vi "Modify JSON Text.vi"(10 "Parameter and Value":string, 11 "JSONtextin":string) -> (3 "JSONtextout":string="{\n    \"SMUResourceName\": \"SMU\",\n    \"SMUChannels\": \"0\",\n\t\"SMUSourceMode_Sequence\": 1021,\n\t\"SMUOutputFunction_DCCurrent\": 1007,\n    \"SMUSourceTransientResponse_Fast\": 1039,\n    \"SMUCurrent\": 1.0,\n    \"SMUCurrentLevelRange\": 1.0,\n    \"SMUMeasurementSense_Local\": 1008,\n    \"SMUMeasurementApertureTime\": 0.010,\n    \"SMUSourceAdvancedSourceDelay\": 0.000100,\n    \"SMUVoltage\": 6,\n    \"SMUSourceAdvancedSequenceLoopCount\": 571,\n    \"SMUMeasurementAdvancedDCNoiseRejection_Normal\": 1044,\n\t\"SMUSequenceName\": \"MySequence\",\n\t\"SMUStep1_Source_DCCurrent_CurrentLevel\": 1150009,\n\t\"SMUStep2_Measurement_ApertureTime\": 1150058,\n\t\"SMUStep3_Source_Advanced_SourceDelay\": 1150051,\n\t\"SMUSequenceNumberOfSteps\": 3,\n\t\"SMUTriggerFromSwitch_StartDigitalEdge\": \"/SMU/PXI_Trig1\",\n\t\"SMUTriggerFromSwitch_SequenceAdvanceDigitalEdge\": \"/SMU/PXI_Trig1\",\n\t\"SMUTriggerToDMM_SourceCompleteEvent\": 1030,\n\t\"SMUTriggerToDMM_SourceCompleteEvent_Value\": \"/SMU/PXI_Trig2\",\n\t\"SMUTriggerToSwitch_SequenceIterationCompleteEvent\": 1032,\n\t\"SMUTriggerToDMM_SequenceIterationCompleteEvent_Value\": \"/SMU/PXI_Trig0\",\n\t\n\t\"Switch1ResourceName\": \"2526_1\",\n\t\"Switch1Topology\": \"2526/2-Wire 79x1 Mux\",\n\t\"Switch1ScanList\": \"ch70:75->com\",\n\t\n\t\"Switch2ResourceName\": \"SwitchBlock1Dev1\",\n\t\"Switch2Topology\": \"Configured Topology\",\n\t\"Switch2ScanList\": \"[c2->card1r2->c26], [c3->card1r3->c27]; [c6->card1r2->c26], [c7->card1r3->c27]; [c10->card1r2->c26], [c11->card1r3->c27]; [c14->card1r2->c26], [c15->card1r3->c27]; [c18->card1r2->c26], [c19->card1r3->c27]; [c22->card1r2->c26], [c23->card1r3->c27];\"\n}")   [LabVIEW 2019]
panel:
  in  "Parameter and Value (for unit testing)":string[](array[string])=["SETCONF=SMUResourceName[[CONFPARAM]]=SMU", "SETCONF=SMUChannels[[CONFPARAM]]=0", "SETCONF=SMUSourceMode_Sequence[[CONFPARAM]]=1021", "SETCONF=SMUOutputFunction_DCCurrent[[CONFPARAM]]=1007", "SETCONF=SMUSourceTransientResponse_Fast[[CONFPARAM]]=1039", "SETCONF=SMUCurrent[[CONFPARAM]]=1.0", "SETCONF=SMUCurrentLevelRange[[CONFPARAM]]=1.0", "SETCONF=SMUMeasurementSense_Local[[CONFPARAM]]=1008", "SETCONF=SMUMeasurementApertureTime[[CONFPARAM]]=0.010", "SETCONF=SMUSourceAdvancedSourceDelay[[CONFPARAM]]=0.000100", "SETCONF=SMUVoltage[[CONFPARAM]]=6", "SETCONF=SMUSourceAdvancedSequenceLoopCount[[CONFPARAM]]=571", "SETCONF=SMUMeasurementAdvancedDCNoiseRejection_Normal[[CONFPARAM]]=1044", "SETCONF=SMUSequenceName[[CONFPARAM]]=MySequence", "SETCONF=SMUStep1_Source_DCCurrent_CurrentLevel[[CONFPARAM]]=1150009", "SETCONF=SMUStep2_Measurement_ApertureTime[[CONFPARAM]]=1150058", "SETCONF=SMUStep3_Source_Advanced_SourceDelay[[CONFPARAM]]=1150051", "SETCONF=SMUSequenceNumberOfSteps[[CONFPARAM]]=3", "SETCONF=SMUTriggerFromSwitch_StartDigitalEdge[[CONFPARAM]]=/SMU/PXI_Trig1", "SETCONF=SMUTriggerFromSwitch_SequenceAdvanceDigitalEdge[[CONFPARAM]]=/SMU/PXI_Trig1", "SETCONF=SMUTriggerToDMM_SourceCompleteEvent[[CONFPARAM]]=1030", "SETCONF=SMUTriggerToDMM_SourceCompleteEvent_Value[[CONFPARAM]]=/SMU/PXI_Trig2", "SETCONF=SMUTriggerToSwitch_SequenceIterationCompleteEvent[[CONFPARAM]]=1032", "SETCONF=SMUTriggerToDMM_SequenceIterationCompleteEvent_Value[[CONFPARAM]]=/SMU/PXI_Trig0", "SETCONF=Switch1ResourceName[[CONFPARAM]]=2526_1", "SETCONF=Switch1Topology[[CONFPARAM]]=2526/2-Wire 79x1 Mux", "SETCONF=Switch1ScanList[[CONFPARAM]]=ch70:75->com", "SETCONF=Switch2ResourceName[[CONFPARAM]]=SwitchBlock1Dev1", "SETCONF=Switch2Topology[[CONFPARAM]]=Configured Topology", "SETCONF=Switch2ScanList[[CONFPARAM]]=[c2->card1r2->c26], [c3->card1r3->c27]; [c6->card1r2->c26], [c7->card1r3->c27]; [c10->card1r2->c26], [c11->card1r3->c27]; [c14->card1r2->c26], [c15->card1r3->c27]; [c18->card1r2->c26], [c19->card1r3->c27]; [c22->card1r2->c26], [c23->card1r3->c27];", "SETCONF=DMMResourceName[[CONFPARAM]]=DMM", "SETCONF=DMMFunction_DCVolts[[CONFPARAM]]=0", "SETCONF=DMMResolution[[CONFPARAM]]=0.1", "SETCONF=DMMRange[[CONFPARAM]]=0.1", "SETCONF=DMMTriggerSource_TTL2[[CONFPARAM]]=4", "SETCONF=DMMTriggerSlope_RisingEdge[[CONFPARAM]]=0", "SETCONF=DMMSampleTrigger_TTL2[[CONFPARAM]]=4", "SETCONF=DMMSampleCount[[CONFPARAM]]=0", "SETCONF=DMMSampleTriggerSlope_RisingEdge[[CONFPARAM]]=0", "SETCONF=DMMApertureTimeUnits_Seconds[[CONFPARAM]]=0", "SETCONF=DMMApertureTime[[CONFPARAM]]=0.010", "SETCONF=DMMNumberOfAverages[[CONFPARAM]]=1", "SETCONF=DMMAutoZero_Off[[CONFPARAM]]=0", "SETCONF=DMMADCCalibration_Off[[CONFPARAM]]=0", "SETCONF=DMMSettleTime[[CONFPARAM]]=0.0001", "SETCONF=DMMControlAction_Commit[[CONFPARAM]]=0", "SETCONF=ApplicationNumberOfWeldChannels[[CONFPARAM]]=6"]
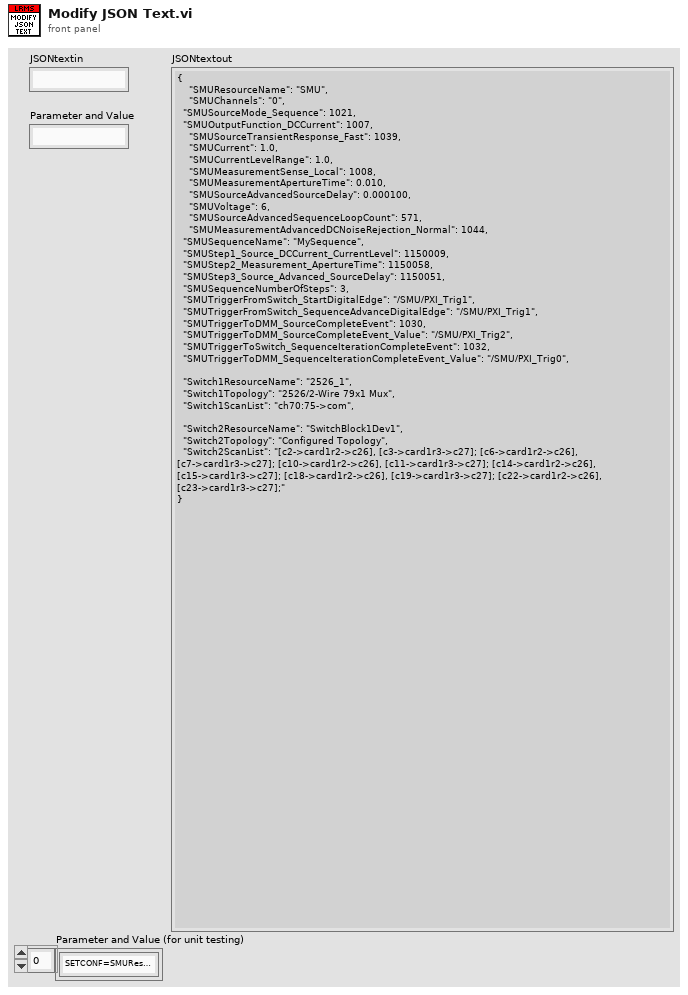
[diagram p1: front panel]
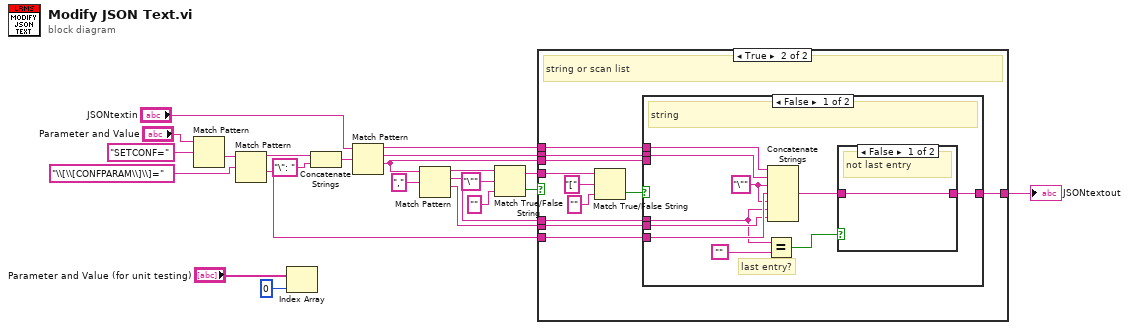
[diagram p0: block diagram]
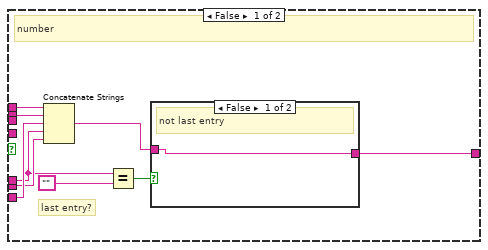
[diagram p2: hidden frame]
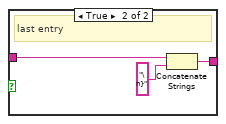
[diagram p3: hidden frame]
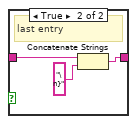
[diagram p4: hidden frame]
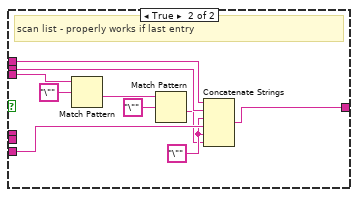
[diagram p5: hidden frame]
diagram:
  n1 = Match Pattern(string="Parameter and Value", regular expression="SETCONF=" ("default value 1")) -> (after substring=w3:string)  [unwired: 1 in, 3 out]
  n2 = Match Pattern(string=w3, regular expression="\\[\\[CONFPARAM\\]\\]=" ("default value 1")) -> (before substring=w6:string, after substring=w15:string)  [unwired: 1 in, 2 out]
  n3 = Index Array(array="Parameter and Value (for unit testing)", index=0) -> ()  [unwired: 1 out]
  n4 = Concatenate Strings(w6, "\": " ("string")) -> (w8:string)
  n5 = Match Pattern(string="JSONtextin", regular expression=w8) -> (before substring=w17:string, match substring=w19:string, after substring=w22:string)  [unwired: 1 in, 1 out]
  n6 = Match Pattern(string=w22, regular expression=",") -> (before substring=w12:string, match substring=w20:string, after substring=w16:string)  [unwired: 1 in, 1 out]
  n7 = Match True/False String(2:"" ("false string"), 3:"\"" ("true string"), 4:w12) -> (0:w13:bool, 1:w21:string)
  n8 = case shown="True" w13 {
    tunnel: w15 -> [w31 w43]
    tunnel: w16 -> [w29 w39]
    tunnel: w17 -> [w32 w42]
    tunnel: [w24 w38] -> w18
    tunnel: w19 -> [w30 w41]
    tunnel: w20 -> [w27 w40]
    tunnel: w21 -> [_ w47]
    tunnel: w22 -> [_ w37]
    frame False {
      # "last entry?"
      # "number"
      n9 = Concatenate Strings(w32, w30, w31, w27, w29) -> (w26:string)
      n10 = Equal?(x=w27, y="") -> (x = y?=w25:bool)
      n11 = case shown="False" w25 {
        tunnel: w26 -> [w33 w36]
        tunnel: [w33 w34] -> w24
        frame False {
          # "not last entry"
        }
        frame True {
          # "last entry"
          n12 = Concatenate Strings(w36, "\n}" ("string")) -> (w34:string)
        }
      }
    }
    frame True {
      # "string or scan list"
      n13 = Match True/False String(2:"" ("false string"), 3:"[" ("true string"), 4:w47) -> (0:w44:bool)  [unwired: 1 out]
      n14 = case shown="False" w44 {
        tunnel: w43 -> [w55 w65]
        tunnel: w42 -> [w57 w67]
        tunnel: w41 -> [w56 w66]
        tunnel: w40 -> [w50 _]
        tunnel: w39 -> [w53 _]
        tunnel: [w48 w63] -> w38
        tunnel: w37 -> [_ w71]
        frame False {
          w54 = "\"" ("string")
          # "last entry?"
          # "string"
          n15 = Equal?(x=w50, y="") -> (x = y?=w51:bool)
          n16 = Concatenate Strings(w57, w56, w54, w55, w54, w50, w53) -> (w49:string)
          n17 = case shown="False" w51 {
            tunnel: w49 -> [w58 w61]
            tunnel: [w58 w59] -> w48
            frame False {
              # "not last entry"
            }
            frame True {
              # "last entry"
              n18 = Concatenate Strings(w61, "\n}" ("string")) -> (w59:string)
            }
          }
        }
        frame True {
          w64 = "\"" ("string")
          # "scan list - properly works if last entry"
          n19 = Match Pattern(string=w71, regular expression="\"") -> (after substring=w69:string)  [unwired: 1 in, 3 out]
          n20 = Match Pattern(string=w69, regular expression="\"") -> (after substring=w62:string)  [unwired: 1 in, 3 out]
          n21 = Concatenate Strings(w67, w66, w64, w65, w64, w62) -> (w63:string)
        }
      }
    }
  }
  "JSONtextout" <- w18
